vi "SubVI_StartDecoder2.vi"(6 "height":u32, 7 "width":u32, 8 "error in":errorcluster, 9 "decoder in":u64, 10 "Destination Image In":T1, 11 "Source Image In":u8[](array[numeric])) -> (0 "error":errorcluster, 1 "elapsed time":u32, 2 "decoder out":u64, 3 "Destination Image Out":T1)   [LabVIEW 2021]
uses:
  <vilib>/vision/Image Controls.llb/IMAQ Image.ctl
  niimaqdx.dll
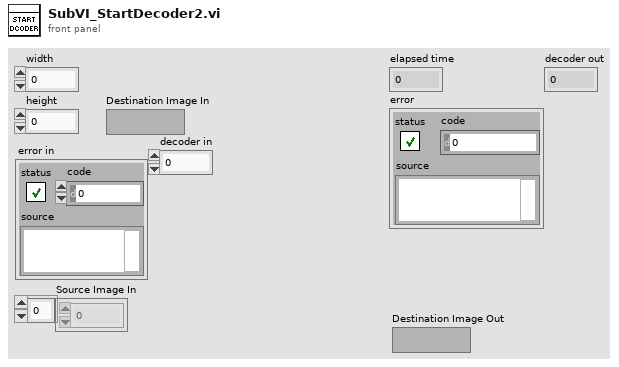
[diagram p1: front panel]
types:
  T1 = typedef "IMAQ Image.ctl" = refnum<image>
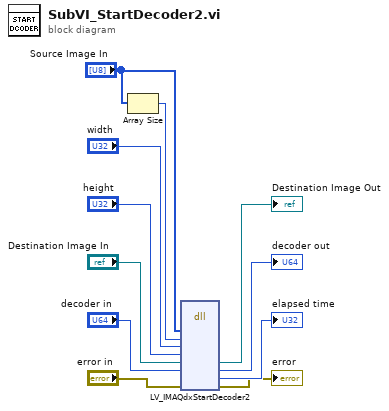
[diagram p0: block diagram]
diagram:
  n1 = Array Size(array="Source Image In") -> (size(s)=w1:i32)
  n2 = dll-call lib="niimaqdx.dll" fn="LV_IMAQdxStartDecoder2"("Source Image"="Source Image In", "imageSizeBytes"=w1, "width"="width", "height"="height", "Destination Image"="Destination Image In", "decoder"="decoder in", "error"="error in") -> ("Destination Image"=→"Destination Image Out":T1, "decoder"=→"decoder out":u64, "elapsed time"=→"elapsed time":u32, "error"=→"error":errorcluster)  [unwired: 4 in, 7 out]
